vi "Create Data Queues.vi"(8 "Error In":errorcluster) -> (0 "Error Out":errorcluster, 3 "Data Queues":T1)   [LabVIEW 2014, in "TDMS Logger.lvlib" / "TDMS Logger.lvclass"]
uses:
  TDMS Logger.lvclass
  _Typedefs/Data Queues.ctl
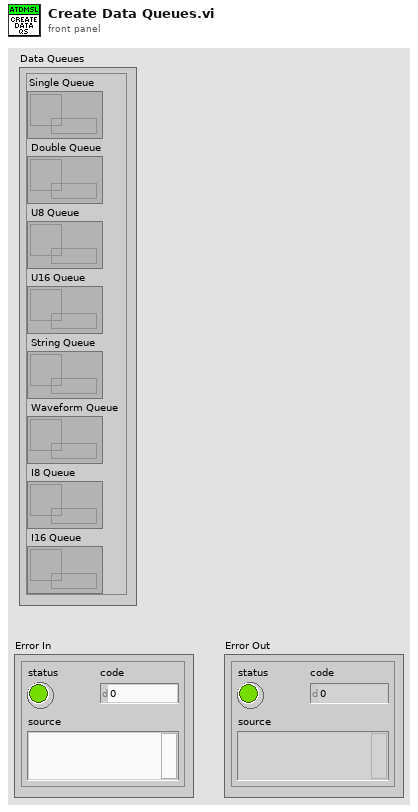
[diagram p1: front panel]
types:
  T1 = typedef "TDMS Logger.lvlib/TDMS Logger.lvclass/Data Queues.ctl" = cluster{"Single Queue":refnum<queue>, "Double Queue":refnum<queue>, "U8 Queue":refnum<queue>, "U16 Queue":refnum<queue>, "String Queue":refnum<queue>, "Waveform Queue":refnum<queue>, "I8 Queue":refnum<queue>, "I16 Queue":refnum<queue>}
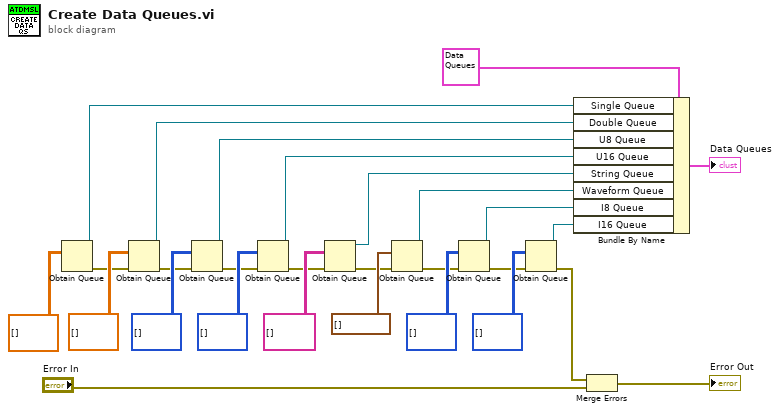
[diagram p0: block diagram]
diagram:
  n1 = Obtain Queue(element data type=sgl[][] [] ("Single")) -> (queue out=w20:refnum<queue>, error out=w1:errorcluster)  [unwired: 4 in, 1 out]
  n2 = Obtain Queue(element data type=dbl[][] [] ("Double"), error in (no error)=w1) -> (queue out=w21:refnum<queue>, error out=w2:errorcluster)  [unwired: 3 in, 1 out]
  n3 = Obtain Queue(element data type=u8[][] [] ("U8"), error in (no error)=w2) -> (queue out=w22:refnum<queue>, error out=w3:errorcluster)  [unwired: 3 in, 1 out]
  n4 = Obtain Queue(element data type=u16[][] [] ("U16"), error in (no error)=w3) -> (queue out=w23:refnum<queue>, error out=w4:errorcluster)  [unwired: 3 in, 1 out]
  n5 = Obtain Queue(element data type=string[][] [], error in (no error)=w4) -> (queue out=w24:refnum<queue>, error out=w5:errorcluster)  [unwired: 3 in, 1 out]
  n6 = Obtain Queue(element data type=waveform(dbl)[] [], error in (no error)=w5) -> (queue out=w25:refnum<queue>, error out=w6:errorcluster)  [unwired: 3 in, 1 out]
  n7 = Obtain Queue(element data type=i8[][] [] ("U8"), error in (no error)=w6) -> (queue out=w26:refnum<queue>, error out=w8:errorcluster)  [unwired: 3 in, 1 out]
  n8 = Obtain Queue(element data type=i16[][] [] ("U8"), error in (no error)=w8) -> (queue out=w27:refnum<queue>, error out=w7:errorcluster)  [unwired: 3 in, 1 out]
  n9 = Bundle By Name(cluster=T1 {"Single Queue"=refnum, "Double Queue"=refnum, "U8 Queue"=refnum, "U16 Queue"=refnum, "String Queue"=refnum, "Waveform Queue"=refnum, "I8 Queue"=refnum, "I16 Queue"=refnum} ("Data Queues"), "Single Queue"=w20, "Double Queue"=w21, "U8 Queue"=w22, "U16 Queue"=w23, "String Queue"=w24, "Waveform Queue"=w25, "I8 Queue"=w26, "I16 Queue"=w27) -> (→"Data Queues":T1)
  n10 = Merge Errors(w7, "Error In") -> (→"Error Out":errorcluster)
